vi "Acquire.vi"(8 "error in (no error)":errorcluster, 11 "TimerSensor in":refnum<class "TimerSensor.lvclass">) -> (0 "error out":errorcluster, 3 "TimerSensor out":refnum<class "TimerSensor.lvclass">)   [LabVIEW 2012, in "TimerSensor.lvlib" / "TimerSensor.lvclass"]
uses:
  TimerSensor.lvclass
  TimerSensorConfig.lvclass
  Sensor Definition/Sensor.lvclass/Sensor.ctl
  Sensor Definition/SensorInfo.lvclass/SensorInfo.ctl
  TimerSensorConfig.lvclass/TimerSensorConfig.ctl
  Sensor Definition/Sensor/Read SensorInfo.vi
  Sensor Definition/Read Config.vi
  TimerSensorConfig/Read Timer Direction.vi
  TimerSensorConfig/Read Target Time.vi
  Sensor Definition/SensorInfo.lvclass
  Sensor Definition/Sensor.lvclass
  Sensor Definition/Double Scalar SensorData.lvclass
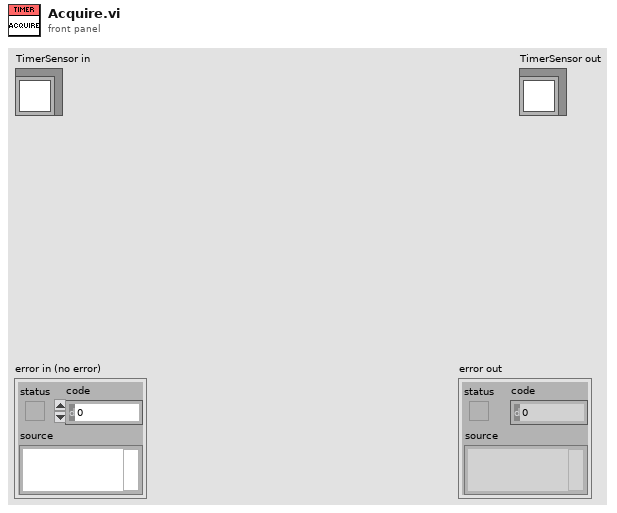
[diagram p1: front panel]
types:
  T1 = typedef "Timer Direction.ctl" = enum16{"Up", "Down"}
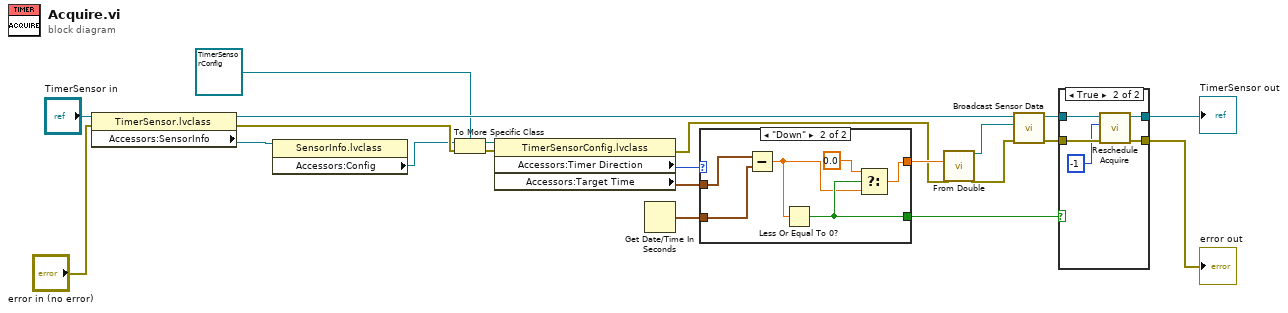
[diagram p0: block diagram]
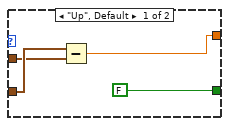
[diagram p3: hidden frame]
diagram:
  n1 = property class="TimerSensor.lvclass"(reference="TimerSensor in", error in="error in (no error)") -> (reference out=w20:refnum<class "TimerSensor.lvclass">, error out=w12:errorcluster, "Accessors:SensorInfo"=w7:refnum<class "SensorInfo.lvclass">)
  n2 = property class="SensorInfo.lvclass"(reference=w7) -> ("Accessors:Config"=w6:refnum<class "SensorConfig.lvclass">)  [unwired: 1 in, 2 out]
  n3 = To More Specific Class(target class=refnum<class "TimerSensorConfig.lvclass"> refnum ("TimerSensor.lvlib:TimerSensorConfig.lvclass"), reference=w6, error in=w12) -> (specific class reference=w15:refnum<class "TimerSensorConfig.lvclass">, error out=w11:errorcluster)
  n4 = property class="TimerSensorConfig.lvclass"(reference=w15, error in=w11) -> (error out=w10:errorcluster, "Accessors:Timer Direction"=w8:T1, "Accessors:Target Time"=w14:timestamp)  [unwired: 1 out]
  n5 = Get Date/Time In Seconds() -> (seconds since 1Jan1904=w19:timestamp)
  n6 = case shown="\"Down\"" w8 {
    tunnel: w19 -> [w25 w31]
    tunnel: [w24 w27] -> w18
    tunnel: w14 -> [w23 w30]
    tunnel: [FALSE w29] -> w1
    frame "Up", Default {
      n7 = Subtract(x=w25, y=w23) -> (x-y=w24:dbl)
    }
    frame "Down" {
      n8 = Subtract(x=w30, y=w31) -> (x-y=w28:dbl)
      n9 = Less Or Equal To 0?(x=w28) -> (x <= 0?=w29:bool)
      n10 = Select(t=0.0, s=w29, f=w28) -> (s? t:f=w27:dbl)
    }
  }
  n11 = call "From Double.vi"("error in (no error)"=w10, "Double"=w18) -> ("error out"=w9:errorcluster, "Double Scalar SensorData out"=w17:refnum<class "Double Scalar SensorData.lvclass">)  [unwired: 8 in]
  n12 = call "Broadcast Sensor Data.vi"("error in (no error)"=w9, "SensorData"=w17, "Sensor in"=w20) -> ("error out"=w3:errorcluster, "Sensor out"=w5:refnum<class "TimerSensor.lvclass">)  [unwired: 7 in]
  n13 = case shown="True" w1 {
    tunnel: w5 -> [w33 w38]
    tunnel: [w33 w37] -> w4
    tunnel: w3 -> [w32 w36]
    tunnel: [w32 w35] -> w2
    frame False {
    }
    frame True {
      n14 = call-dynamic "Reschedule Acquire.vi"("error in (no error)"=w36, "Sample Time"=-1, "Sensor in"=w38) -> ("error out"=w35:errorcluster, "Sensor out"=w37:refnum<class "TimerSensor.lvclass">)  [unwired: 7 in]
    }
  }
  "error out" <- w2
  "TimerSensor out" <- w4
